vi "InitializeApplicationPaths.vi"(8 "error in (no error)":errorcluster) -> (0 "error out":errorcluster)   [LabVIEW 2011]
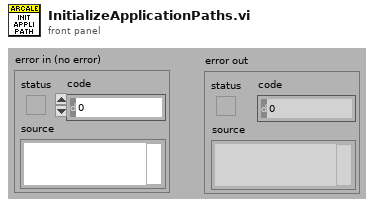
[diagram p1: front panel]
types:
  T1 = typedef "ApplicationPaths.ctl" = cluster{"Data Path":path, "Log Path":path, "Tmp Path":path}
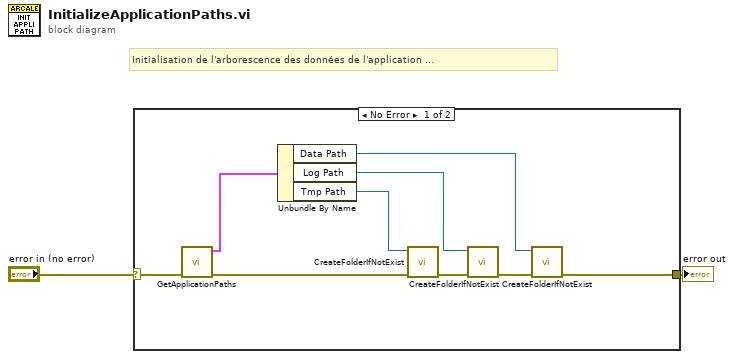
[diagram p0: block diagram]
diagram:
  # "Initialisation de l'arborescence des données de l'application ..."
  n1 = case shown="No Error" "error in (no error)" {
    selector: "error in (no error)" -> [w11 w12]
    tunnel: [w5 w12] -> w1
    frame No Error {
      n2 = call "GetApplicationPaths.vi"("error in (no error)"=w11) -> ("error out"=w3:errorcluster, "ApplicationPath"=w10:T1)  [unwired: 9 in]
      n3 = Unbundle By Name(w10) -> ("Data Path"=w4:path, "Log Path"=w7:path, "Tmp Path"=w9:path)
      n4 = call "CreateFolderIfNotExist.vi"("errorIn"=w3, "Data Path"=w9) -> ("error out"=w8:errorcluster)  [unwired: 9 in]
      n5 = call "CreateFolderIfNotExist.vi"("errorIn"=w8, "Data Path"=w7) -> ("error out"=w6:errorcluster)  [unwired: 9 in]
      n6 = call "CreateFolderIfNotExist.vi"("errorIn"=w6, "Data Path"=w4) -> ("error out"=w5:errorcluster)  [unwired: 9 in]
    }
    frame Error {
    }
  }
  "error out" <- w1
